vi "Show Caller Items Dialog.vi"(6 "Event":refnum<vi>, 8 "Find Broadcast?":bool=TRUE, 11 "Request VI Callers":refnum<vi>[](array[refnum])) -> ()   [LabVIEW 2020, in "Panther Dashboard.lvlib"]
uses:
  Panther Dashboard.lvlib
  Controls/MulticolumListbox.ctl
panel:
  in  "Open All":bool
  in  "Results Listbox":T1
  # "» Double click an element to navigate in the callercode\n» Right-click an item to browse the file on disk"
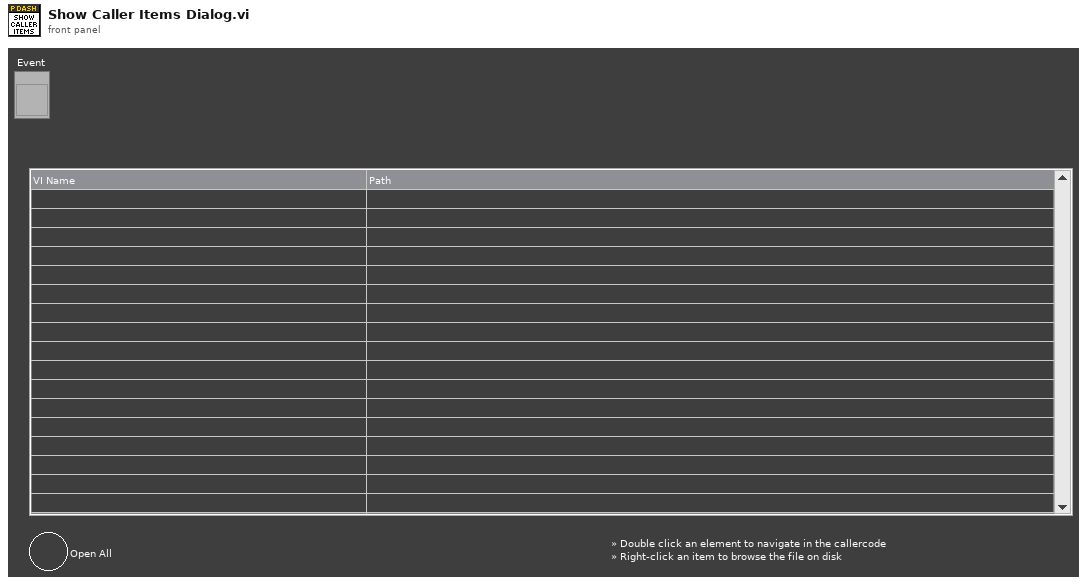
[diagram p1: front panel]
types:
  T1 = typedef "MulticolumListbox.ctl" = i32
  T2 = typedef "LVRowAndColumnTypeDef.ctl" = cluster{"Row":i32, "Column":i32}
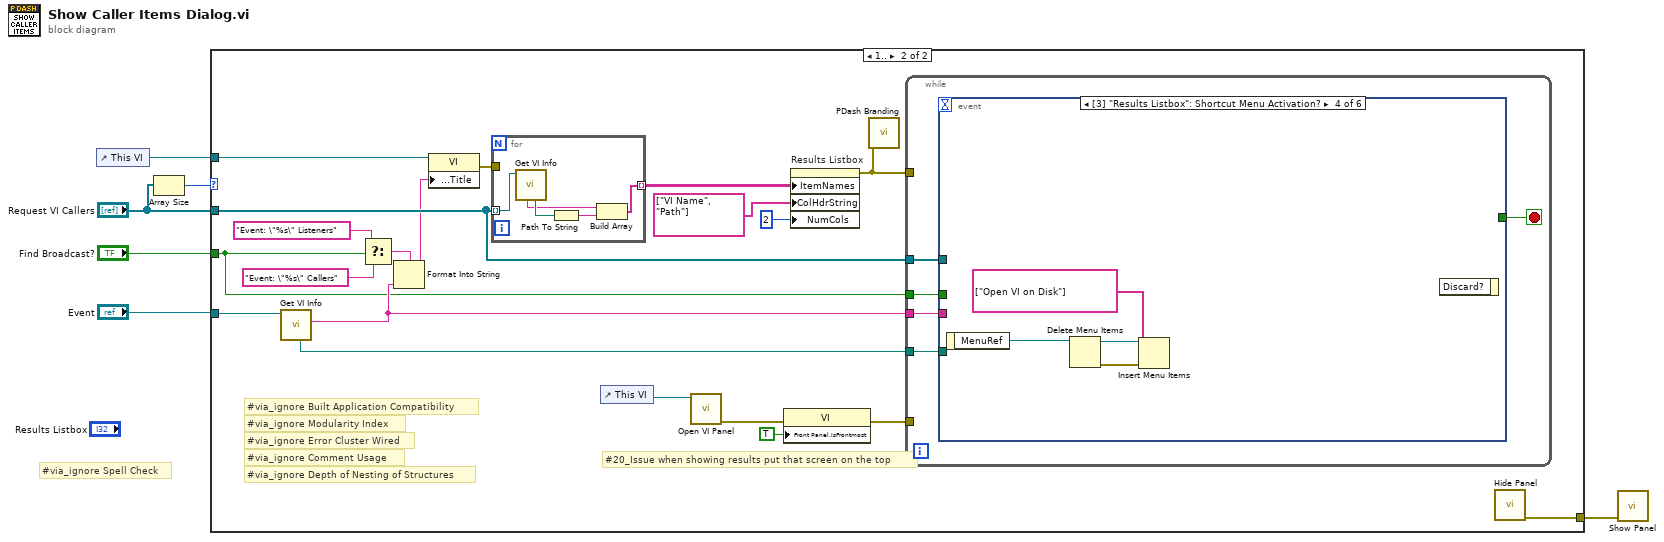
[diagram p0: block diagram]
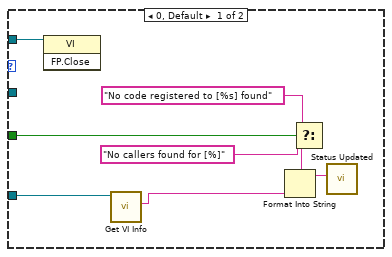
[diagram p2: hidden frame]
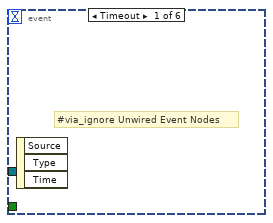
[diagram p3: hidden frame]
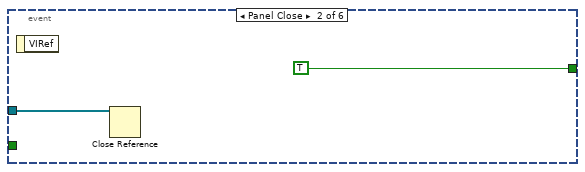
[diagram p4: hidden frame]
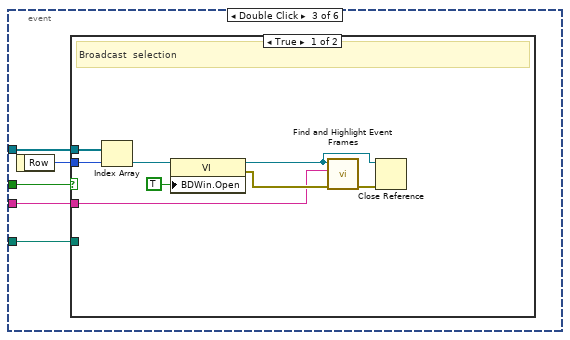
[diagram p5: hidden frame]
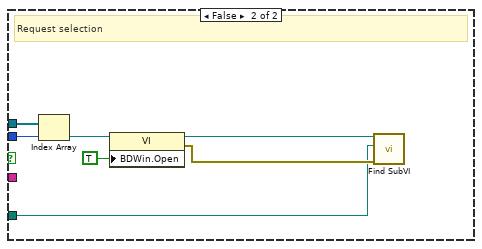
[diagram p6: hidden frame]
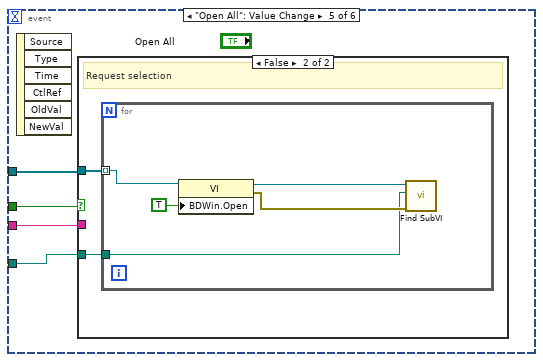
[diagram p7: hidden frame]
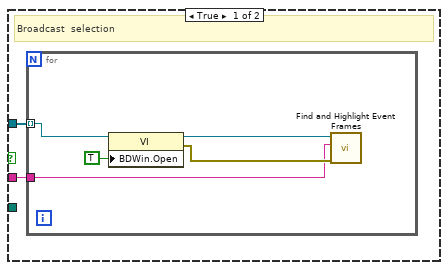
[diagram p8: hidden frame]
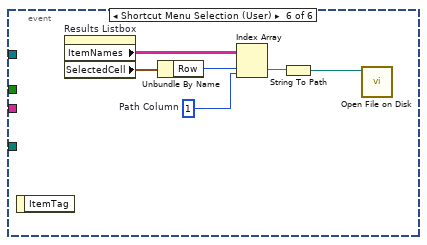
[diagram p9: hidden frame]
diagram:
  # "#via_ignore Spell Check"
  n1 = control-ref of="This VI"() -> (w2:refnum<vi>)
  n2 = Array Size(array="Request VI Callers") -> (size(s)=w5:i32)
  n3 = case shown="1.." w5 {
    tunnel: "Request VI Callers" -> [_ w27]
    tunnel: "Event" -> [w8 w26]
    tunnel: "Find Broadcast?" -> [w13 w19]
    tunnel: w2 -> [w9 w24]
    tunnel: [_ w22] -> w1
    frame 0, Default {
      n4 = invoke class="VI" method="FP.Close"(reference=w9) -> ()  [unwired: 2 in, 3 out]
      n5 = call "Get VI Info.vi"("VI in"=w8) -> ("Plain Name"=w7:string)  [unwired: 5 in, 5 out]
      n6 = Select(t="No code registered to [%s] found" ("Origin"), s=w13, f="No callers found for [%]" ("Origin")) -> (s? t:f=w11:string)
      n7 = Format Into String(format string=w11, w7) -> (resulting string=w14:string)  [unwired: 2 in, 1 out]
      n8 = call "Status Updated.vi"("Status"=w14) -> ()  [unwired: 10 in, 1 out]
    }
    frame 1.. {
      # "#20_Issue when showing results put that screen on the top"
      # "#via_ignore Built Application Compatibility"
      # "#via_ignore Modularity Index"
      # "#via_ignore Depth of Nesting of Structures"
      # "#via_ignore Error Cluster Wired"
      # "#via_ignore Comment Usage"
      n9 = call "Get VI Info.vi"("VI in"=w26) -> ("Plain Name"=w25:string, "VI Path"=w18:path)  [unwired: 5 in, 4 out]
      n10 = Select(t="Event: \"%s\" Listeners" ("Origin"), s=w19, f="Event: \"%s\" Callers" ("Origin")) -> (s? t:f=w29:string)
      n11 = Format Into String(format string=w29, w25) -> (resulting string=w23:string)  [unwired: 2 in, 1 out]
      n12 = property class="VI"(reference=w24, "Front Panel.Title"=w23) -> (error out=w34:errorcluster)  [unwired: 1 in, 1 out]
      n13 = for {
        tunnel: w27 -> [w37] mode=indexing
        tunnel: [w38] -> w33 mode=indexing
        tunnel: w34 -> [_]
        n14 = call "Get VI Info.vi"("VI in"=w37) -> ("VI Path"=w36:path, "VI Name"=w35:string)  [unwired: 5 in, 4 out]
        n15 = Path To String(path=w36) -> (string=w39:string)
        n16 = Build Array(w35, w39) -> (w38:string[])
      }
      n17 = control-ref of="This VI"() -> (w16:refnum<vi>)
      n18 = call "Open VI Panel.vi"("VI"=w16) -> ("error out"=w17:errorcluster)  [unwired: 10 in]
      n19 = property class="VI"(error in=w17, "Front Panel.IsFrontmost"=TRUE ("Front Panel Window:Is Frontmost")) -> (error out=w21:errorcluster)  [unwired: 1 in, 1 out]
      n20 = property on="Results Listbox" class="MCListbox (strict)"("ItemNames"=w33, "ColHdrString"=string[] ["VI Name", "Path"] ("Column Header Strings[]"), "NumCols"=u32 2 ("Number of Columns")) -> (error out=w15:errorcluster)  [unwired: 2 in, 1 out]
      n21 = call "PDash Branding.vi"("error in"=w15) -> ()  [unwired: 11 in]
      n22 = while {
        tunnel: w27 -> [w44]
        tunnel: w15 -> [_]
        tunnel: w19 -> [w42]
        tunnel: w25 -> [w41]
        tunnel: w21 -> [_]
        tunnel: w18 -> [w40]
        stop <- w43 stop-if-true
        n23 = event shown="[3] \"Results Listbox\": Shortcut Menu Activation?" {
          selector: _ -> [_ _ _ _ _ _]
          dyn-events: _ -> [_ _ _ _ _ _]
          timeout: _ -> [_ _ _ _ _ _]
          tunnel: w44 -> [_ w46 w51 _ w74 _]
          tunnel: [_ TRUE _ _ _ _] -> w43
          tunnel: w42 -> [_ _ w49 _ w72 _]
          tunnel: w41 -> [_ _ w48 _ w73 _]
          tunnel: w40 -> [_ _ w47 _ w71 _]
          event Timeout {
            # "#via_ignore Unwired Event Nodes"
            n24 = event-data() -> ()  [unwired: 1 in, 3 out]
          }
          event Panel Close {
            n25 = event-data() -> ()  [unwired: 1 in, 1 out]
            n26 = Close Reference(reference=w46) -> ()  [unwired: 1 in, 1 out]
          }
          event Double Click {
            n27 = event-data() -> ("Row"=w50:i32)  [unwired: 1 in]
            n28 = case shown="True" w49 {
              tunnel: w51 -> [w58 w65]
              tunnel: w50 -> [w57 w64]
              tunnel: w48 -> [w53 _]
              tunnel: w47 -> [_ w60]
              frame True {
                # "Broadcast  selection"
                n29 = Index Array(array=w58, index=w57) -> (element=w56:refnum<vi>)
                n30 = property class="VI"(reference=w56, "BDWin.Open"=TRUE ("Block Diagram Window:Open")) -> (reference out=w52:refnum<vi>, error out=w55:errorcluster)  [unwired: 1 in]
                n31 = call "Find and Highlight Event Frames.vi"("error in"=w55, "Event Name"=w53, "VI Reference"=w52) -> ("error out"=w54:errorcluster)  [unwired: 7 in, 1 out]
                n32 = Close Reference(reference=w52, error in (no error)=w54) -> ()  [unwired: 1 out]
              }
              frame False {
                # "Request selection"
                n33 = Index Array(array=w65, index=w64) -> (element=w63:refnum<vi>)
                n34 = property class="VI"(reference=w63, "BDWin.Open"=TRUE ("Block Diagram Window:Open")) -> (reference out=w61:refnum<vi>, error out=w62:errorcluster)  [unwired: 1 in]
                n35 = call "Find SubVI.vi"("error in"=w62, "VI Path"=w60, "VI Reference"=w61) -> ()  [unwired: 7 in, 2 out]
              }
            }
          }
          event Shortcut Menu Activation? {
            n36 = event-data() -> ("MenuRef"=w70:refnum<k9>)  [unwired: 1 in]
            n37 = Delete Menu Items(9:w70) -> (0:w68:errorcluster, 3:w69:refnum<k9>)  [unwired: 3 in]
            n38 = Insert Menu Items(6:w68, 8:string[] ["Open VI on Disk"] ("item names"), 9:w69) -> ()  [unwired: 3 in, 3 out]
            n39 = event-data() -> ()  [unwired: 2 in, 1 out]
          }
          event "Open All": Value Change {
            n40 = event-data() -> ()  [unwired: 1 in, 6 out]
            n41 = case shown="False" w72 {
              tunnel: w74 -> [w76 w83]
              tunnel: w73 -> [w75 _]
              tunnel: w71 -> [_ w82]
              frame True {
                # "Broadcast  selection"
                n42 = for {
                  tunnel: w76 -> [w79] mode=indexing
                  tunnel: w75 -> [w77]
                  n43 = property class="VI"(reference=w79, "BDWin.Open"=TRUE ("Block Diagram Window:Open")) -> (reference out=w78:refnum<vi>, error out=w80:errorcluster)  [unwired: 1 in]
                  n44 = call "Find and Highlight Event Frames.vi"("error in"=w80, "Event Name"=w77, "VI Reference"=w78) -> ()  [unwired: 7 in, 2 out]
                }
              }
              frame False {
                # "Request selection"
                n45 = for {
                  tunnel: w83 -> [w86] mode=indexing
                  tunnel: w82 -> [w84]
                  n46 = property class="VI"(reference=w86, "BDWin.Open"=TRUE ("Block Diagram Window:Open")) -> (reference out=w85:refnum<vi>, error out=w87:errorcluster)  [unwired: 1 in]
                  n47 = call "Find SubVI.vi"("error in"=w87, "VI Path"=w84, "VI Reference"=w85) -> ()  [unwired: 7 in, 2 out]
                }
              }
            }
          }
          event Shortcut Menu Selection (User) {
            w91 = 1  # Path Column
            n48 = event-data() -> ()  [unwired: 1 in, 1 out]
            n49 = property on="Results Listbox" class="MCListbox (strict)"() -> ("ItemNames"=w94:string[][], "SelectedCell"=w93:T2)  [unwired: 2 in, 2 out]
            n50 = Unbundle By Name(w93) -> ("Row"=w92:i32)
            n51 = Index Array(array=w94, index (row)=w92, index (col)=w91) -> (element=w90:string)
            n52 = String To Path(string=w90) -> (path=w89:path)
            n53 = call "Open File on Disk.vi"("file or directory path"=w89) -> ()  [unwired: 10 in, 1 out]
          }
        }
      }
      n54 = call "Hide Panel.vi"() -> ("error out"=w22:errorcluster)  [unwired: 11 in]
    }
  }
  n55 = call "Show Panel.vi"("error in (no error)"=w1) -> ()  [unwired: 10 in, 1 out]
